vi "task1.vi"() -> ()   [LabVIEW 2020]
panel:
  out "Number of iterations":i64
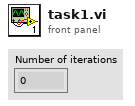
[diagram p1: front panel]
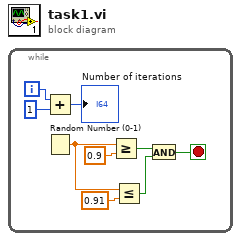
[diagram p0: block diagram]
diagram:
  n1 = while {
    i -> [w3]
    stop <- w5 stop-if-true
    n2 = Add(x=w3, y=1) -> (x+y=→"Number of iterations":i32)
    n3 = Random Number (0-1)() -> (number: 0 to 1=w4:dbl)
    n4 = Greater Or Equal?(x=w4, y=0.9) -> (x >= y?=w9:bool)
    n5 = Less Or Equal?(x=w4, y=0.91) -> (x <= y?=w6:bool)
    n6 = And(x=w9, y=w6) -> (x .and. y?=w5:bool)
  }
